vi "Handle Error.vi"(8 "error in (no error)":errorcluster caption="错误输入（无错误）", 11 "EPEVER-MPPT in":refnum<class "EPEVER-MPPT.lvclass"> caption="操作者输入") -> (0 "error out":errorcluster caption="错误输出", 2 "stop actor?":bool=TRUE caption="停止操作者？", 3 "EPEVER-MPPT out":refnum<class "EPEVER-MPPT.lvclass"> caption="操作者输出")   [LabVIEW 2016, in "EPEVER-MPPT.lvlib" / "EPEVER-MPPT.lvclass"]
doc: "(<B>Filename</B>: Actor Framework.lvlib:Actor.lvclass:Handle Error.vi)\n\nDefines how the actor handles an error that occurred while processing a message.默认情况下，该方法不执行任何操作，仅停止操作者。"
uses:
  EPEVER-MPPT.lvclass
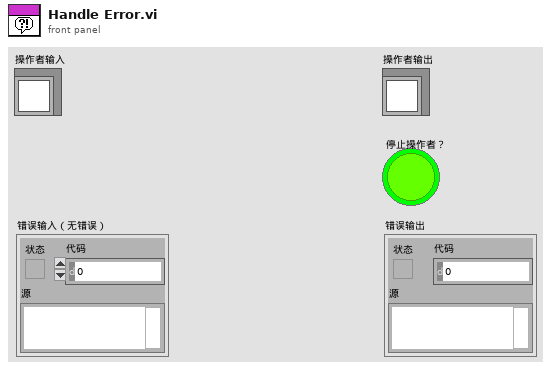
[diagram p1: front panel]
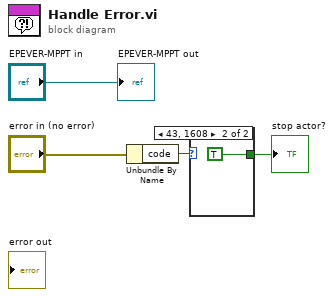
[diagram p0: block diagram]
diagram:
  n1 = Unbundle By Name("error in (no error)") -> ("code"=w3:i32)
  n2 = case shown="43, 1608" w3 {
    tunnel: [_ TRUE] -> w4
    frame 0, Default {
    }
    frame 43, 1608 {
    }
  }
  "stop actor?" <- w4
  "EPEVER-MPPT out" <- "EPEVER-MPPT in"
